vi "Default Settings.vi"(8 "error in (no error)":errorcluster, 11 "C4 Dispense in 2":refnum<class "Iterative Dispense.lvclass">) -> (0 "error out":errorcluster, 3 "C4 Dispense out 2":refnum<class "Iterative Dispense.lvclass">)   [LabVIEW 2020, in "Iterative Dispense.lvclass"]
uses:
  Iterative Dispense.lvclass
  C:/Users/hep/Documents/CMU gantry/Classes/Routine/Dispense/Dispense.lvclass
  Iterative Dispense.lvclass/Iterative Dispense.ctl
  Dispense.lvclass/Dispense.ctl
  Write Tip Height.vi
panel:
  # "This Routine does not Accept Settings"
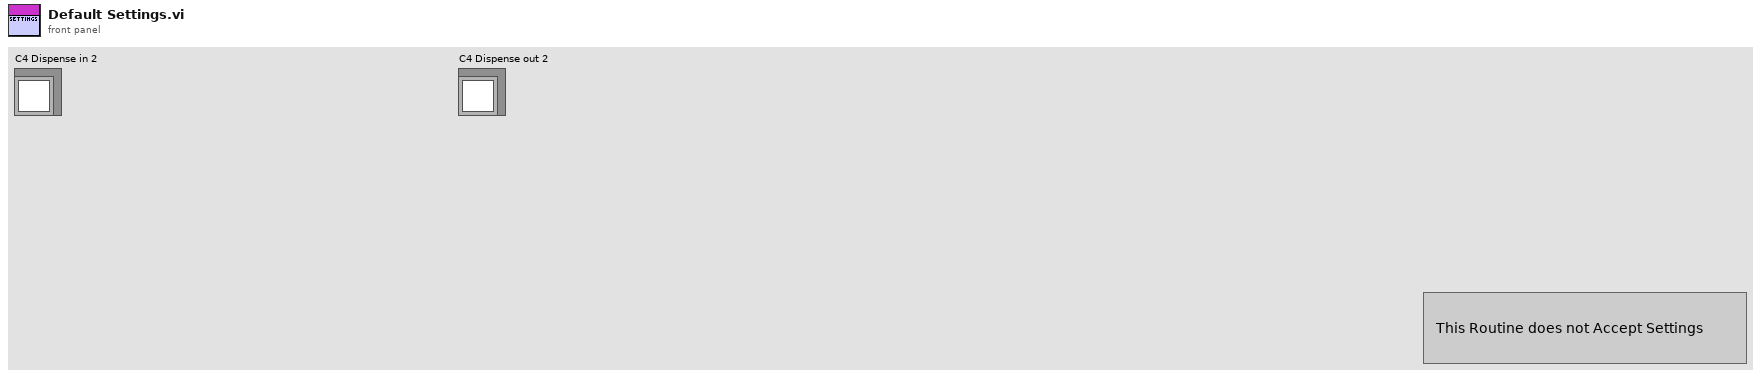
[diagram p1: front panel]
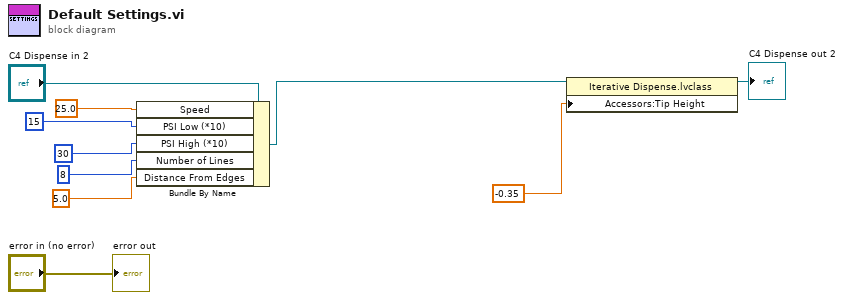
[diagram p0: block diagram]
diagram:
  n1 = Bundle By Name(cluster="C4 Dispense in 2", "Speed"=25.0, "PSI Low (*10)"=15, "PSI High (*10)"=30, "Number of Lines"=8 ("Lines"), "Distance From Edges"=5.0 ("Edge Distance")) -> (w1:refnum<class "Iterative Dispense.lvclass">)
  n2 = property class="Iterative Dispense.lvclass"(reference=w1, "Accessors:Tip Height"=-0.35 ("Tip Height")) -> (reference out=→"C4 Dispense out 2":refnum<class "Iterative Dispense.lvclass">)  [unwired: 1 in, 1 out]
  "error out" <- "error in (no error)"
